vi "begincvlib.vi"(8 "error in (no error)":errorcluster, 10 "backend":u32(ring) items=["USEBEST", "CUDA", "OPENCL"], 11 "ClearVolumeJarPath":string) -> (0 "error out":errorcluster, 2 "function return":u32, 3 "ClearVolumeJarPath out":string)   [LabVIEW 2012, in "clearvolume.lvlib"]
doc: "__declspec(dllexport) unsigned long __cdecl begincvlib(char* ClearVolumeJarPath, backend_t backend);"
uses:
  clearvolume.lvlib
  clearvolume.dll
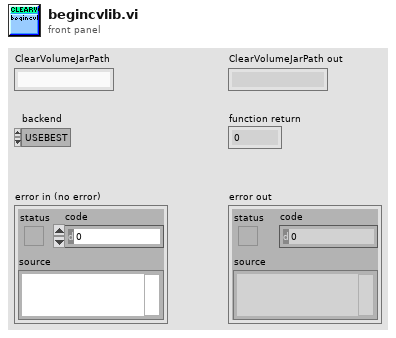
[diagram p1: front panel]
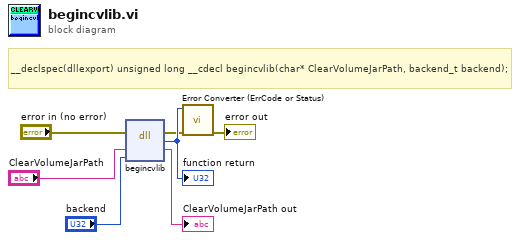
[diagram p0: block diagram]
diagram:
  # "__declspec(dllexport) unsigned long __cdecl begincvlib(char* ClearVolumeJarPath, backend_t backend);"
  n1 = dll-call lib="C:/Users/myerslab/workspace/Libraries/CV/clearvolume/src/labview/clearvolume/clearvolume.*" fn="begincvlib"(error in="error in (no error)", "ClearVolumeJarPath"="ClearVolumeJarPath", "backend"="backend") -> (error out=w2:errorcluster, w7:u32, "ClearVolumeJarPath"=→"ClearVolumeJarPath out":string)  [unwired: 3 in, 1 out]
  "function return" <- w7
  n2 = call "Error Converter (ErrCode or Status).vi"("error in (no error)"=w2, "error code"=w7) -> ("error out"=→"error out":errorcluster)  [unwired: 9 in]
